vi "Show Scales Read.vi"(4 "error in (no error)":errorcluster, 6 "Container State":T2, 7 "Display State In":T1) -> (0 "error out":errorcluster, 2 "Value":bool, 3 "Display State Out":T1)   [LabVIEW 2011, in "Waveform Control.xctl"]
doc: "Show scales property determines whether the azes labels are shown on the graphical display of the waveform."
uses:
  Waveform Control.xctl
  <vilib>/_xctls/Container State.ctl
  Controls/State.ctl
  Controls/Volatile State Ops.ctl
  <vilib>/_xctls/XControlSupport.lvlib
panel:
  # "Replace the Value Indicator below with an Indicator of desired type.\nDo not remove this Indicator or the others from the connector pane. \nDo not change the connector pane pattern.\nThe Value Indicator should always be the second terminal from top on the output side in the connector pane."
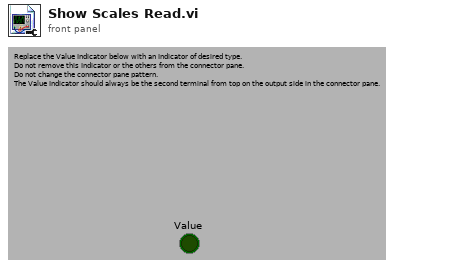
[diagram p1: front panel]
types:
  T1 = typedef "Waveform Control.xctl/State.ctl" = cluster{"Name":string}
  T2 = typedef "XControlSupport.lvlib/Container State.ctl" = cluster{"Indicator?":bool, "Run Mode?":bool, " Refnum":refnum<vi>}
  T3 = typedef "Waveform Control.xctl/Volatile State Ops.ctl" = enum16{"Read", "Write", "Update State from Data"}
  T4 = typedef "Waveform Control.xctl/Waveform State.ctl" = cluster{"Show Axes":bool, "Show Y=0":bool, "Controls":T5, "Show Current Location":bool, "Current Location":i32, "dt":dbl, "t0":timestamp}
  T5 = typedef "Waveform Control.xctl/FP Controls.ctl" = cluster{"Type":T6, "Periods":dbl, "Points":i32, "Offset":dbl, "Amplitdue":dbl, "Starting Phase":dbl, "func":string}
  T6 = typedef "Waveform Control.xctl/Function Types.ctl" = enum16{"Level", "Sine", "Triangle", "Ramp", "Saw Tooth", "Square", "Function"}
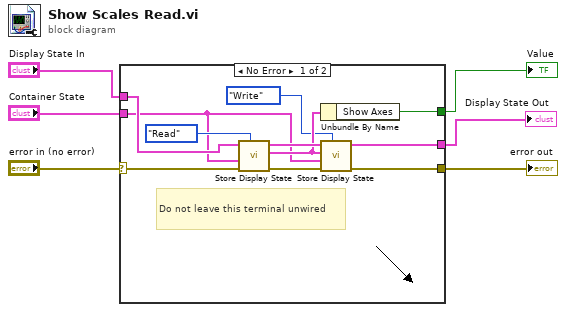
[diagram p0: block diagram]
diagram:
  n1 = case shown="No Error" "error in (no error)" {
    selector: "error in (no error)" -> [w15 w19]
    tunnel: "Display State In" -> [w17 w18]
    tunnel: [w14 w19] -> w4
    tunnel: [w9 _] -> w3
    tunnel: [w8 w18] -> w2
    tunnel: "Container State" -> [w7 _]
    frame No Error {
      # "Do not leave this terminal unwired"
      n2 = call "Store Display State.vi"("Operation In"=Volatile_State_Ops."Read" ("Operation"), "Error In (no Error) In"=w15, "Container State In"=w7, "State In"=w17) -> ("Error Out"=w16:errorcluster, "Waveform State Out"=w12:T4, "Display State Out"=w13:T1)  [unwired: 2 in, 3 out]
      n3 = Unbundle By Name(w12) -> ("Show Axes"=w9:bool)
      n4 = call "Store Display State.vi"("Operation In"=Volatile_State_Ops."Write" ("Operation"), "Error In (no Error) In"=w16, "Container State In"=w7, "Waveform State In"=w12, "State In"=w13) -> ("Error Out"=w14:errorcluster, "Display State Out"=w8:T1)  [unwired: 1 in, 4 out]
    }
    frame Error {
    }
  }
  "error out" <- w4
  "Value" <- w3
  "Display State Out" <- w2
